vi "updateValues.vi"(8 "error in (no error)":errorcluster, 11 "Rf_Ramp_Action in":refnum<class "Rf_Ramp_Action.lvclass">) -> (0 "error out":errorcluster, 3 "Rf_Ramp_Action out":refnum<class "Rf_Ramp_Action.lvclass">)   [LabVIEW 2009, in "Views.lvlib" / "ScriptEditor.lvlib" / "Rf_Ramp_Action.lvclass"]
uses:
  Rf_Ramp_Action.lvclass
  Tools/Scripting/ScriptingEvent/ScriptEvents/RfRamp/RfRamp.lvclass
  Rf_Ramp_Action.lvclass/Rf_Ramp_Action.ctl
  Tools/Scripting/ScriptingEvent/ScriptEvent.lvclass
  Tools/Scripting/ScriptingEvent/ScriptEvents/Rf Event/rf.lvclass
  ActionPanel.lvclass
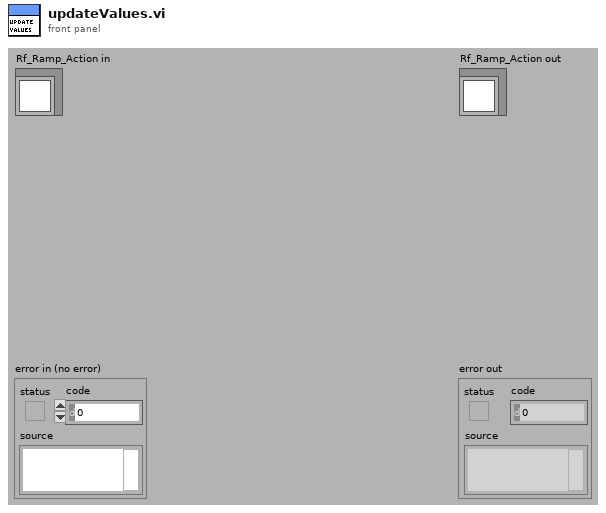
[diagram p1: front panel]
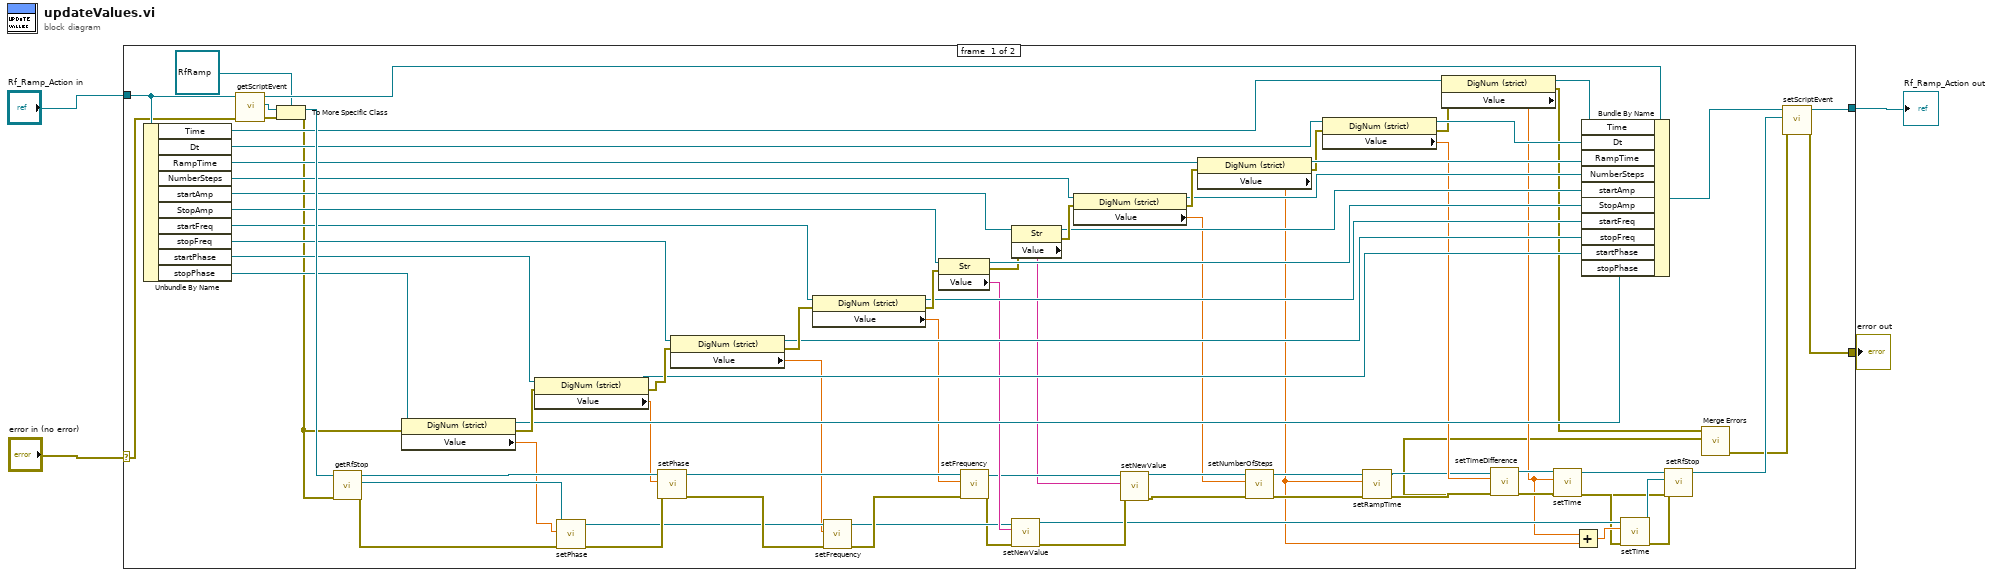
[diagram p0: block diagram]
diagram:
  n1 = case shown="No Error" "error in (no error)" {
    selector: "error in (no error)" -> [w83 w86]
    tunnel: [w6 w86] -> w3
    tunnel: [w8 w85] -> w1
    tunnel: "Rf_Ramp_Action in" -> [w84 w85]
    frame #0 {
      n2 = Unbundle By Name(w84) -> ("Time"=w50:refnum<vi>, "Dt"=w53:refnum<vi>, "RampTime"=w55:refnum<vi>, "NumberSteps"=w56:refnum<vi>, "startAmp"=w58:refnum<vi>, "StopAmp"=w61:refnum<vi>, "startFreq"=w62:refnum<vi>, "stopFreq"=w63:refnum<vi>, "startPhase"=w64:refnum<vi>, "stopPhase"=w65:refnum<vi>)
      n3 = call "getScriptEvent.vi"("error in (no error)"=w83, "ActionPanel.lvclass in"=w84) -> ("error out"=w67:errorcluster, "ScriptEvent.lvclass"=w69:refnum<class "ScriptEvent.lvclass">, "ActionPanel.lvclass out"=w70:refnum<class "Rf_Ramp_Action.lvclass">)  [unwired: 7 in]
      n4 = To More Specific Class(target class=refnum<class "RfRamp.lvclass"> refnum ("RfRamp out"), reference=w69, error in=w67) -> (specific class reference=w66:refnum<class "RfRamp.lvclass">, error out=w44:errorcluster)
      n5 = call "getRfStop.vi"("error in (no error)"=w44, "RfRamp in"=w66) -> ("error out"=w45:errorcluster, "rfStop"=w49:refnum<class "rf.lvclass">, "RfRamp out"=w48:refnum<class "RfRamp.lvclass">)  [unwired: 7 in]
      n6 = property class="DigNum (strict)"(reference=w65, error in=w44) -> (reference out=w71:refnum<vi>, error out=w72:errorcluster, "Value"=w5:dbl)
      n7 = property class="DigNum (strict)"(reference=w64, error in=w72) -> (reference out=w73:refnum<vi>, error out=w82:errorcluster, "Value"=w47:dbl)
      n8 = call "setPhase.vi"("error in (no error)"=w45, "phase"=w5, "rf in"=w49) -> ("error out"=w46:errorcluster, "rf out"=w40:refnum<class "rf.lvclass">)  [unwired: 7 in]
      n9 = call "setPhase.vi"("error in (no error)"=w46, "phase"=w47, "rf in"=w48) -> ("error out"=w41:errorcluster, "rf out"=w43:refnum<class "RfRamp.lvclass">)  [unwired: 7 in]
      n10 = property class="DigNum (strict)"(reference=w63, error in=w82) -> (reference out=w74:refnum<vi>, error out=w81:errorcluster, "Value"=w39:dbl)
      n11 = property class="DigNum (strict)"(reference=w62, error in=w81) -> (reference out=w75:refnum<vi>, error out=w80:errorcluster, "Value"=w38:dbl)
      n12 = call "setFrequency.vi"("error in (no error)"=w41, "frequency"=w39, "rf in"=w40) -> ("error out"=w42:errorcluster, "rf out"=w36:refnum<class "rf.lvclass">)  [unwired: 7 in]
      n13 = property class="Str"(reference=w61, error in=w80) -> (reference out=w76:refnum<vi>, error out=w59:errorcluster, "Value"=w37:string)
      n14 = call "setFrequency.vi"("error in (no error)"=w42, "frequency"=w38, "rf in"=w43) -> ("error out"=w35:errorcluster, "rf out"=w34:refnum<class "RfRamp.lvclass">)  [unwired: 7 in]
      n15 = property class="Str"(reference=w58, error in=w59) -> (reference out=w57:refnum<vi>, error out=w60:errorcluster, "Value"=w32:string)
      n16 = call "setNewValue.vi"("error in (no error)"=w35, "newValue"=w37, "ScriptEvent.lvclass in"=w36) -> ("error out"=w33:errorcluster, "ScriptEvent.lvclass out"=w20:refnum<class "rf.lvclass">)  [unwired: 7 in]
      n17 = property class="DigNum (strict)"(reference=w56, error in=w60) -> (reference out=w77:refnum<vi>, error out=w79:errorcluster, "Value"=w30:dbl)
      n18 = call "setNewValue.vi"("error in (no error)"=w33, "newValue"=w32, "ScriptEvent.lvclass in"=w34) -> ("error out"=w29:errorcluster, "ScriptEvent.lvclass out"=w31:refnum<class "RfRamp.lvclass">)  [unwired: 7 in]
      n19 = property class="DigNum (strict)"(reference=w55, error in=w79) -> (reference out=w78:refnum<vi>, error out=w54:errorcluster, "Value"=w18:dbl)
      n20 = call "setNumberOfSteps.vi"("error in (no error)"=w29, "NumberOfSteps"=w30, "RfRamp in"=w31) -> ("error out"=w27:errorcluster, "RfRamp out"=w28:refnum<class "RfRamp.lvclass">)  [unwired: 7 in]
      n21 = property class="DigNum (strict)"(reference=w53, error in=w54) -> (reference out=w52:refnum<vi>, error out=w25:errorcluster, "Value"=w26:dbl)
      n22 = call "setRampTime.vi"("error in (no error)"=w27, "rampTime"=w18, "RfRamp in"=w28) -> ("error out"=w15:errorcluster, "RfRamp out"=w16:refnum<class "RfRamp.lvclass">)  [unwired: 7 in]
      n23 = property class="DigNum (strict)"(reference=w50, error in=w25) -> (reference out=w51:refnum<vi>, error out=w22:errorcluster, "Value"=w19:dbl)
      n24 = call "setTimeDifference.vi"("error in (no error)"=w15, "time difference"=w26, "ScriptEvent.lvclass in"=w16) -> ("error out"=w23:errorcluster, "ScriptEvent.lvclass out"=w24:refnum<class "RfRamp.lvclass">)  [unwired: 7 in]
      n25 = call "setTime.vi"("error in (no error)"=w23, "time"=w19, "ScriptEvent.lvclass in"=w24) -> ("error out"=w17:errorcluster, "ScriptEvent.lvclass out"=w14:refnum<class "RfRamp.lvclass">)  [unwired: 7 in]
      n26 = Add(x=w19, y=w18) -> (x+y=w21:dbl)
      n27 = Bundle By Name(cluster=w70, "Time"=w51, "Dt"=w52, "RampTime"=w78, "NumberSteps"=w77, "startAmp"=w57, "StopAmp"=w76, "startFreq"=w75, "stopFreq"=w74, "startPhase"=w73, "stopPhase"=w71) -> (w10:refnum<class "Rf_Ramp_Action.lvclass">)
      n28 = call "setTime.vi"("error in (no error)"=w17, "time"=w21, "ScriptEvent.lvclass in"=w20) -> ("error out"=w12:errorcluster, "ScriptEvent.lvclass out"=w13:refnum<class "rf.lvclass">)  [unwired: 7 in]
      n29 = call "setRfStop.vi"("error in (no error)"=w12, "rfStop"=w13, "RfRamp in"=w14) -> ("error out"=w11:errorcluster, "RfRamp out"=w9:refnum<class "RfRamp.lvclass">)  [unwired: 7 in]
      n30 = call <vilib>:"Merge Errors.vi"("error in 2 (no error)"=w11, "error in 1 (no error)"=w22) -> ("error out"=w7:errorcluster)  [unwired: 5 in]
      n31 = call "setScriptEvent.vi"("error in (no error)"=w7, "ScriptEvent.lvclass"=w9, "ActionPanel.lvclass in"=w10) -> ("error out"=w6:errorcluster, "ActionPanel.lvclass out"=w8:refnum<class "Rf_Ramp_Action.lvclass">)  [unwired: 7 in]
    }
    frame #1 {
    }
  }
  "error out" <- w3
  "Rf_Ramp_Action out" <- w1
